vi "rmad event to file.vi"(0 "Skredhendelser":T2(array[cluster]) {"Intensitet terskel 1" format="%.1f"; "Intensitet terskel 2" format="%.1f"; "Intensitet terskel 3" format="%.1f"; "Intensitet terskel 4" format="%.1f"; "Intensitet terskel 5" format="%.1f"}, 1 "vdv_datadir":string, 3 "event_datadir":string, 7 "Recent events 2":T1(array[cluster]) {"SPS" format="%.1f"}, 9 "last packet type":u8[](array[numeric]), 11 "error in":errorcluster, 12 "event to file?":bool[](array[boolean]), 13 "mac adresses":T3) -> (15 "error out":errorcluster)   [LabVIEW 2017]
panel:
  out "previous line in dat file":string
  out "last vdv record number":i32
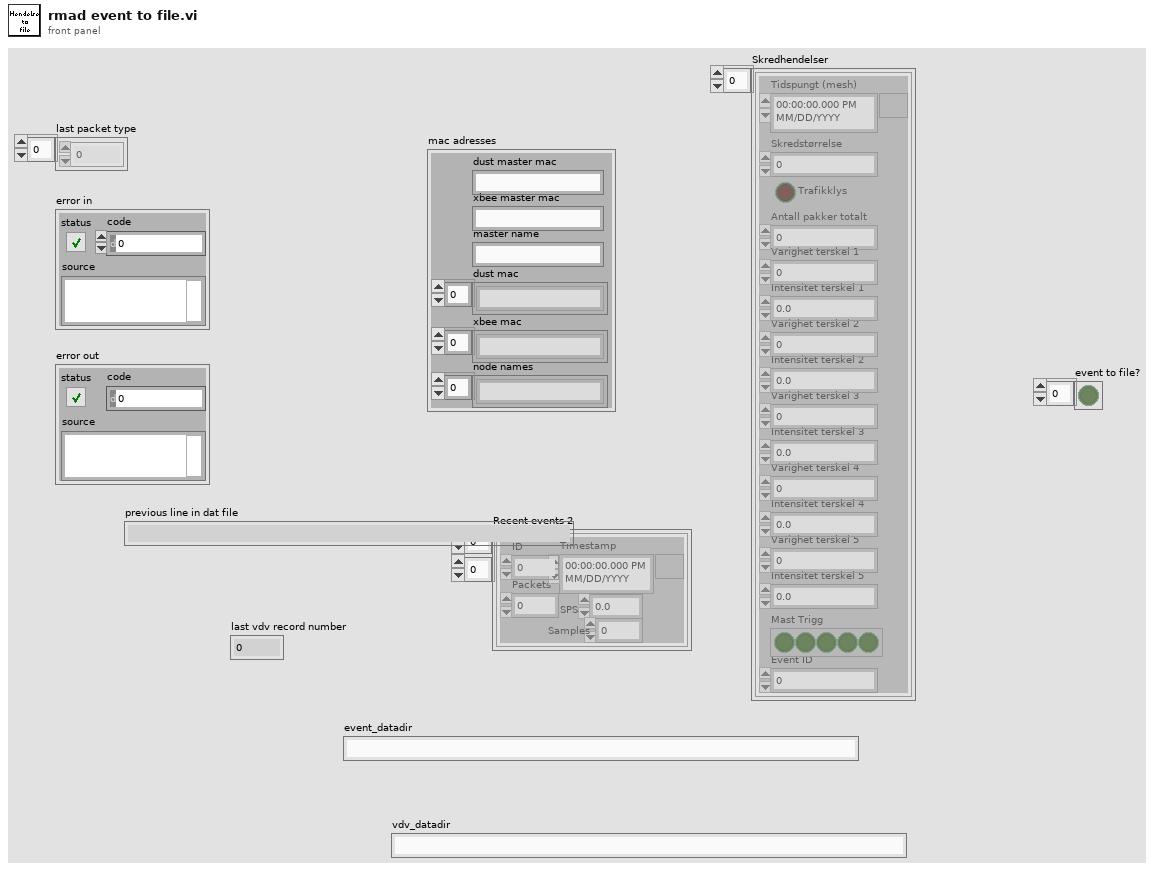
[diagram p1: front panel]
types:
  T1 = cluster{"ID":u16, "Timestamp":timestamp, "Packets":u16, "SPS":dbl, "Samples":u16}[][]
  T2 = cluster{"Tidspungt (mesh)":timestamp, "Skredstørrelse":u16, "Trafikklys":bool, "Antall pakker totalt":u16, "Varighet terskel 1":u16, "Intensitet terskel 1":dbl, "Varighet terskel 2":u16, "Intensitet terskel 2":dbl, "Varighet terskel 3":u16, "Intensitet terskel 3":dbl, "Varighet terskel 4":u16, "Intensitet terskel 4":dbl, "Varighet terskel 5":u16, "Intensitet terskel 5":dbl, "Mast Trigg":bool[], "Event ID":i32}[]
  T3 = cluster{"dust master mac":string, "xbee master mac":string, "master name":string, "dust mac":string[], "xbee mac":string[], "node names":string[]}
  T4 = enum16{"open", "replace", "create", "open or create", "replace or create", "replace or create with confirmation"}
  T5 = cluster{"ID":u16, "Timestamp":timestamp, "Packets":u16, "SPS":dbl, "Samples":u16}
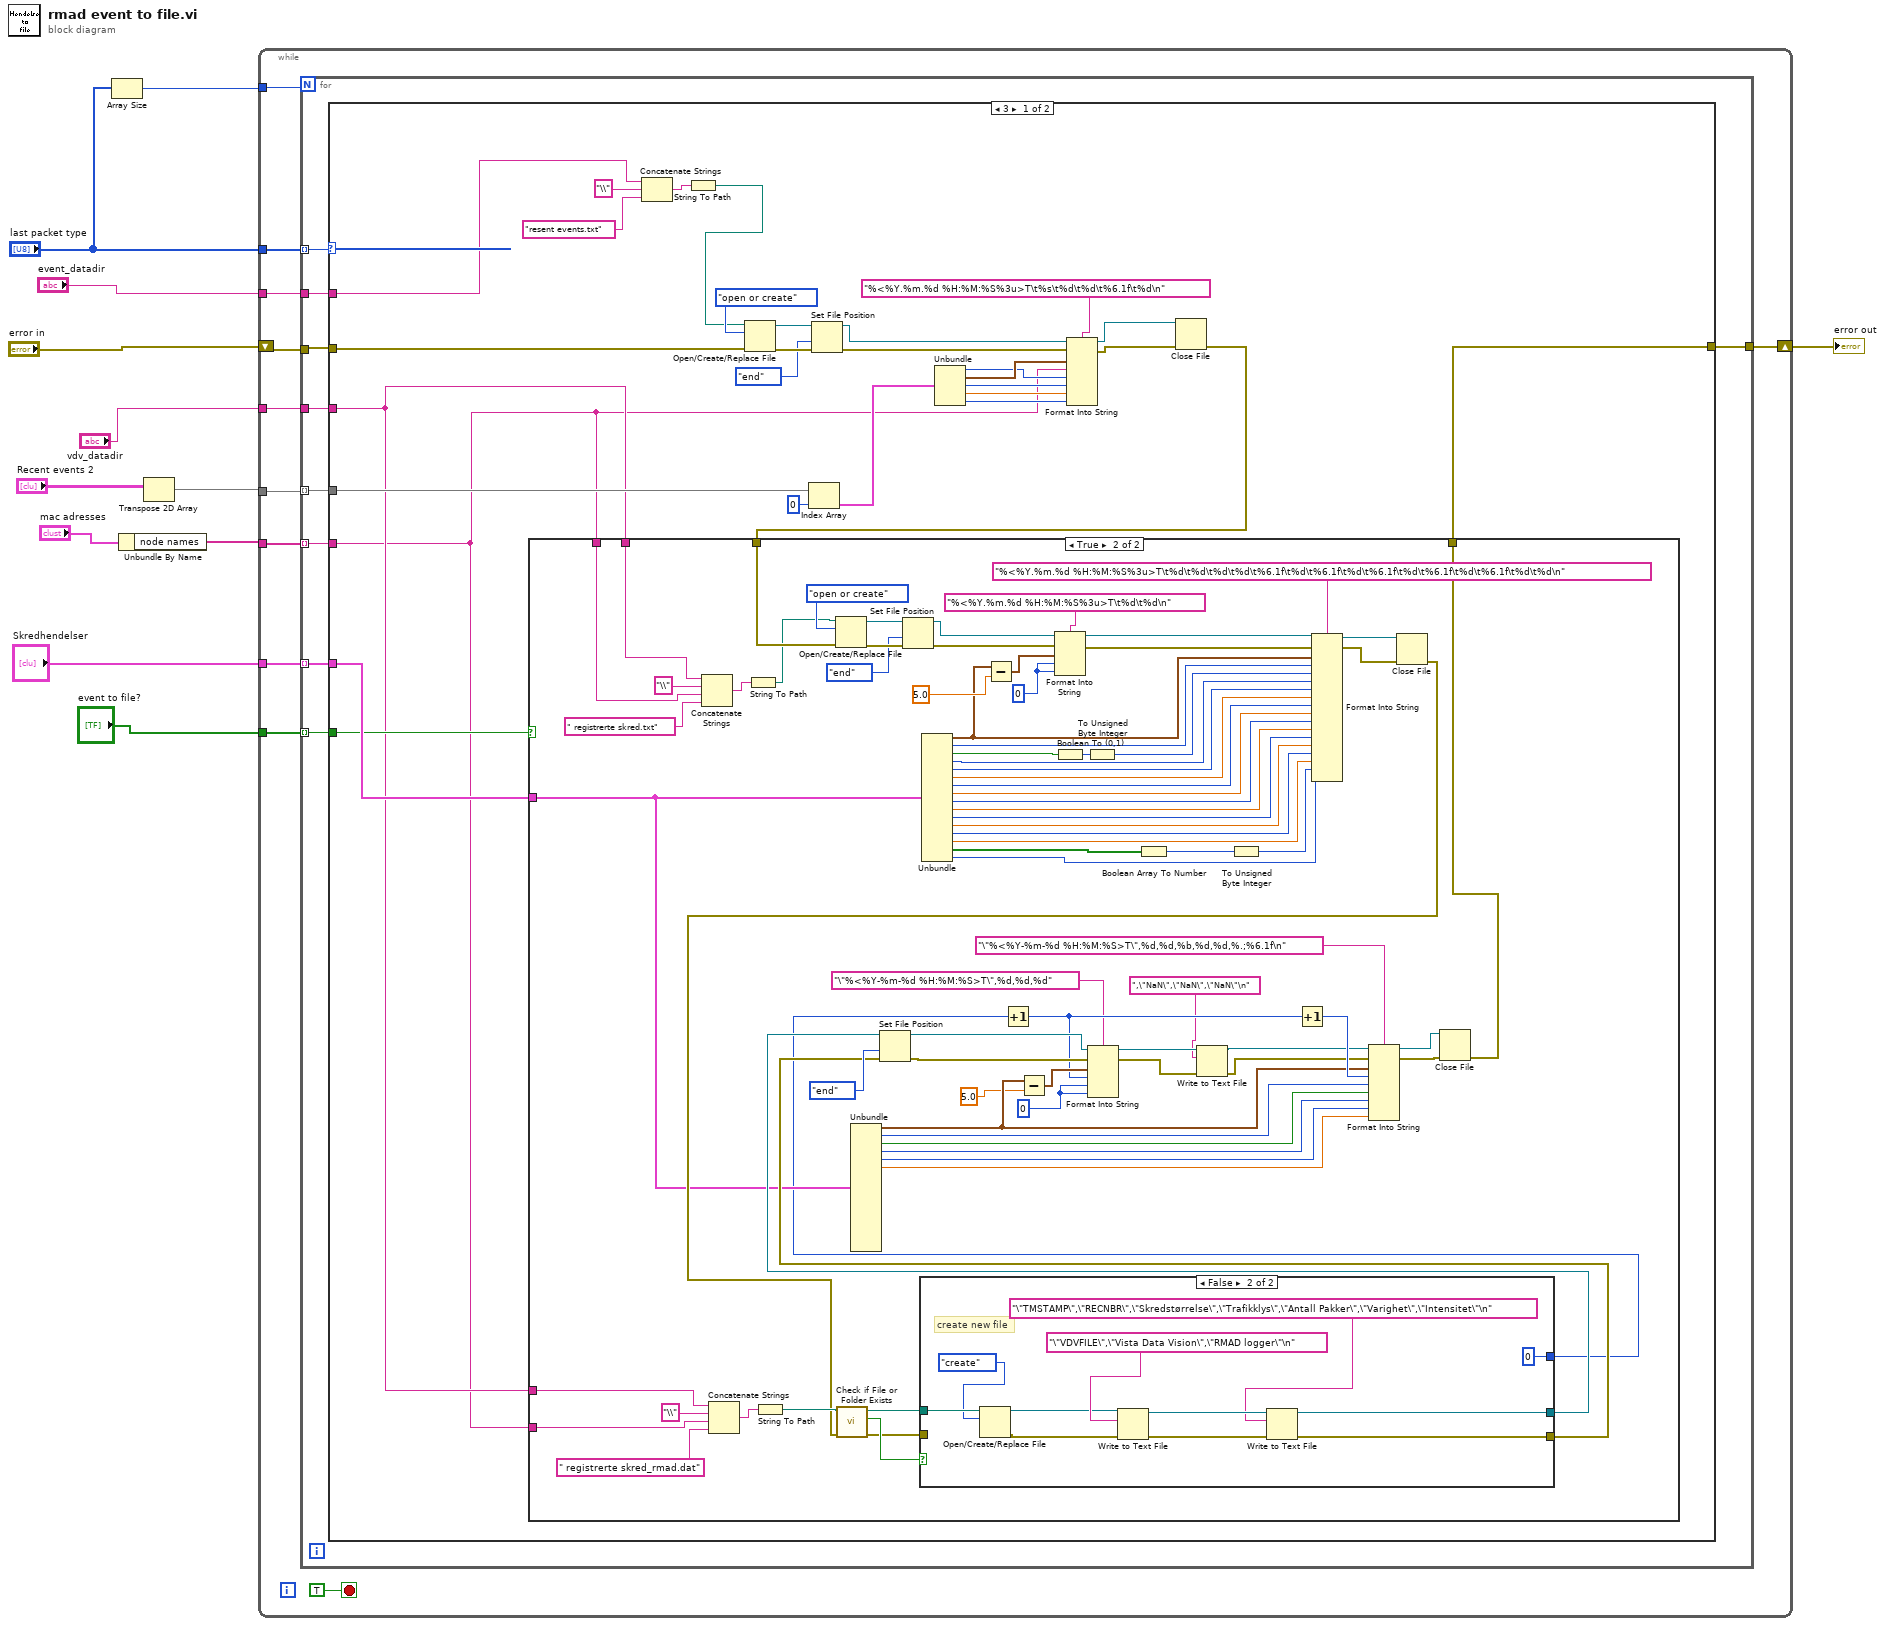
[diagram p0: block diagram]
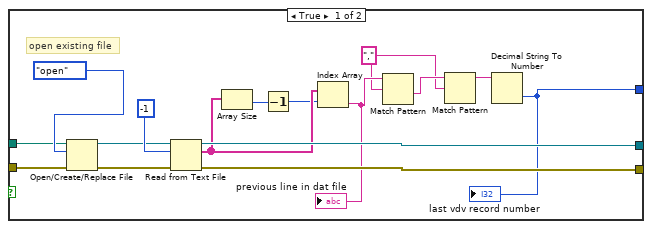
[diagram p3: hidden frame]
diagram:
  n1 = Array Size(array="last packet type") -> (size(s)=w9:i32)
  n2 = Unbundle By Name("mac adresses") -> ("node names"=w6:string[])
  n3 = Transpose 2D Array(2D array="Recent events 2") -> (transposed array=w5:T1)
  n4 = while {
    tunnel: "event_datadir" -> [w21]
    tunnel: w9 -> [w16]
    tunnel: "last packet type" -> [w20]
    tunnel: w6 -> [w19]
    tunnel: w5 -> [w18]
    shift-right: [w22] -> w11
    shift-left: "error in" -> [w23]
    tunnel: "Skredhendelser" -> [w15]
    tunnel: "vdv_datadir" -> [w14]
    tunnel: "event to file?" -> [w13]
    stop <- TRUE stop-if-true
    n5 = for {
      N: w16 -> [_]
      tunnel: w20 -> [w32] mode=indexing
      tunnel: w23 -> [w31]
      tunnel: [w26] -> w22
      tunnel: w21 -> [w30]
      tunnel: w19 -> [w28] mode=indexing
      tunnel: w18 -> [w29] mode=indexing
      tunnel: w15 -> [w27] mode=indexing
      tunnel: w14 -> [w25]
      tunnel: w13 -> [w24] mode=indexing
      n6 = case shown="3" w32 {
        tunnel: w31 -> [w61 w170]
        tunnel: [w39 w170] -> w26
        tunnel: w30 -> [w38 _]
        tunnel: w28 -> [w33 _]
        tunnel: w29 -> [w52 _]
        tunnel: w27 -> [w37 _]
        tunnel: w25 -> [w34 _]
        tunnel: w24 -> [w35 _]
        frame 3 {
          n7 = Concatenate Strings(w38, "\\" ("string"), "resent events.txt" ("string")) -> (w55:string)
          n8 = String To Path(string=w55) -> (path=w54:path)
          n9 = Open/Create/Replace File(file path (use dialog)=w54, error in=w61, operation (0:open)=T4."open or create") -> (refnum out=w58:refnum<file>, error out=w59:errorcluster)  [unwired: 3 in, 1 out]
          n10 = Index Array(array=w52, index=0) -> (element=w50:T5)
          n11 = Set File Position(refnum=w58, from (0:start)=enum16{"start", "end", "current"}."end", error in=w59) -> (refnum out=w43:refnum<file>, error out=w45:errorcluster)  [unwired: 1 in]
          n12 = Unbundle(w50) -> ("ID"=w40:u16, "Timestamp"=w49:timestamp, "Packets"=w48:u16, "SPS"=w36:dbl, "Samples"=w47:u16)
          n13 = Format Into String(format string="%<%Y.%m.%d %H:%M:%S%3u>T\t%s\t%d\t%d\t%6.1f\t%d\n", initial string=w43, error in=w45, w49, w33, w40, w48, w36, w47) -> (resulting string=w42:refnum<file>, error out=w44:errorcluster)
          n14 = Close File(refnum=w42, error in=w44) -> (error out=w41:errorcluster)  [unwired: 1 out]
          n15 = case shown="True" w35 {
            tunnel: w41 -> [w62 w138]
            tunnel: [w62 w83] -> w39
            tunnel: w34 -> [_ w134]
            tunnel: w33 -> [_ w133]
            tunnel: w37 -> [_ w82]
            tunnel: w34 -> [_ w86]
            tunnel: w33 -> [_ w85]
            frame False {
            }
            frame True {
              w71 = u8 0 ("input 2")
              w105 = u8 0 ("input 2")
              n16 = Concatenate Strings(w134, "\\" ("string"), w133, " registrerte skred.txt" ("string")) -> (w136:string)
              n17 = Concatenate Strings(w86, "\\" ("string"), w85, " registrerte skred_rmad.dat" ("string")) -> (w97:string)
              n18 = String To Path(string=w136) -> (path=w132:path)
              n19 = String To Path(string=w97) -> (path=w91:path)
              n20 = Open/Create/Replace File(file path (use dialog)=w132, error in=w138, operation (0:open)=T4."open or create") -> (refnum out=w140:refnum<file>, error out=w141:errorcluster)  [unwired: 3 in, 1 out]
              n21 = Unbundle(w82) -> ("Tidspungt (mesh)"=w73:timestamp, "Skredstørrelse"=w81:u16, "Trafikklys"=w88:bool, "Antall pakker totalt"=w89:u16, "Varighet terskel 1"=w80:u16, "Intensitet terskel 1"=w79:dbl)  [unwired: 10 out]
              n22 = Set File Position(refnum=w140, from (0:start)=enum16{"start", "end", "current"}."end", error in=w141) -> (refnum out=w126:refnum<file>, error out=w128:errorcluster)  [unwired: 1 in]
              n23 = Unbundle(w82) -> ("Tidspungt (mesh)"=w120:timestamp, "Skredstørrelse"=w121:u16, "Trafikklys"=w103:bool, "Antall pakker totalt"=w117:u16, "Varighet terskel 1"=w116:u16, "Intensitet terskel 1"=w115:dbl, "Varighet terskel 2"=w114:u16, "Intensitet terskel 2"=w113:dbl, "Varighet terskel 3"=w112:u16, "Intensitet terskel 3"=w111:dbl, "Varighet terskel 4"=w110:u16, "Intensitet terskel 4"=w109:dbl, "Varighet terskel 5"=w108:u16, "Intensitet terskel 5"=w107:dbl, "Mast Trigg"=w102:bool[], "Event ID"=w104:i32)
              n24 = Subtract(x=w120, y=5.0) -> (x-y=w123:timestamp)
              n25 = Subtract(x=w73, y=5.0) -> (x-y=w76:timestamp)
              n26 = Format Into String(format string="%<%Y.%m.%d %H:%M:%S%3u>T\t%d\t%d\n", initial string=w126, error in=w128, w123, w105, w105) -> (resulting string=w125:refnum<file>, error out=w127:errorcluster)
              n27 = Boolean To (0,1)(Boolean=w103) -> (0, 1=w118:i16)
              n28 = To Unsigned Byte Integer(number=w118) -> (unsigned 8bit integer=w119:u8)
              n29 = Boolean Array To Number(Boolean array=w102) -> (number=w101:u32)
              n30 = To Unsigned Byte Integer(number=w101) -> (unsigned 8bit integer=w106:u8)
              n31 = Format Into String(format string="%<%Y.%m.%d %H:%M:%S%3u>T\t%d\t%d\t%d\t%d\t%6.1f\t%d\t%6.1f\t%d\t%6.1f\t%d\t%6.1f\t%d\t%6.1f\t%d\t%d\n", initial string=w125, error in=w127, w120, w121, w119, w117, w116, w115, w114, w113, w112, w111, w110, w109, w108, w107, w106, w104) -> (resulting string=w129:refnum<file>, error out=w130:errorcluster)
              n32 = Close File(refnum=w129, error in=w130) -> (error out=w84:errorcluster)  [unwired: 1 out]
              n33 = call <vilib>:"Check if File or Folder Exists.vi"("error in (no error)"=w84, "path"=w91) -> ("error out"=w94:errorcluster, "file or folder exists?"=w95:bool, "dup path"=w90:path)  [unwired: 7 in]
              n34 = case shown="False" w95 {
                tunnel: w90 -> [w156 w169]
                tunnel: [w155 w161] -> w93
                tunnel: [w154 w160] -> w92
                tunnel: w94 -> [w158 _]
                tunnel: [w143 0] -> w70
                frame True {
                  w145 = "," ("regular expression")
                  # "open existing file"
                  n35 = Open/Create/Replace File(file path (use dialog)=w156, error in=w158, operation (0:open)=T4."open") -> (refnum out=w151:refnum<file>, error out=w152:errorcluster)  [unwired: 3 in, 1 out]
                  n36 = Read from Text File(file (use dialog)=w151, count=-1, error in=w152) -> (refnum out=w154:refnum<file>, text=w150:string[], error out=w155:errorcluster)  [unwired: 1 in, 1 out]
                  n37 = Array Size(array=w150) -> (size(s)=w149:i32)
                  n38 = Decrement(x=w149) -> (x-1=w148:i32)
                  n39 = Index Array(array=w150, index=w148) -> (element=w147:string)
                  "previous line in dat file" <- w147
                  n40 = Match Pattern(string=w147, regular expression=w145) -> (after substring=w146:string)  [unwired: 1 in, 3 out]
                  n41 = Match Pattern(string=w146, regular expression=w145) -> (before substring=w144:string)  [unwired: 1 in, 3 out]
                  n42 = Decimal String To Number(string=w144) -> (number=w143:i32)  [unwired: 2 in, 1 out]
                  "last vdv record number" <- w143
                }
                frame False {
                  # "create new file"
                  n43 = Open/Create/Replace File(file path (use dialog)=w169, operation (0:open)=T4."create") -> (refnum out=w165:refnum<file>, error out=w166:errorcluster)  [unwired: 4 in, 1 out]
                  n44 = Write to Text File(file (use dialog)=w165, text="\"VDVFILE\",\"Vista Data Vision\",\"RMAD logger\"\n" ("format string"), error in=w166) -> (refnum out=w163:refnum<file>, error out=w164:errorcluster)  [unwired: 1 in, 1 out]
                  n45 = Write to Text File(file (use dialog)=w163, text="\"TMSTAMP\",\"RECNBR\",\"Skredstørrelse\",\"Trafikklys\",\"Antall Pakker\",\"Varighet\",\"Intensitet\"\n" ("format string"), error in=w164) -> (refnum out=w160:refnum<file>, error out=w161:errorcluster)  [unwired: 1 in, 1 out]
                }
              }
              n46 = Set File Position(refnum=w92, from (0:start)=enum16{"start", "end", "current"}."end", error in=w93) -> (refnum out=w74:refnum<file>, error out=w75:errorcluster)  [unwired: 1 in]
              n47 = Increment(x=w70) -> (x+1=w69:i32)
              n48 = Format Into String(format string="\"%<%Y-%m-%d %H:%M:%S>T\",%d,%d,%d", initial string=w74, error in=w75, w76, w69, w71, w71) -> (resulting string=w67:refnum<file>, error out=w65:errorcluster)
              n49 = Write to Text File(file (use dialog)=w67, text=",\"NaN\",\"NaN\",\"NaN\"\n", error in=w65) -> (refnum out=w66:refnum<file>, error out=w64:errorcluster)  [unwired: 1 in, 1 out]
              n50 = Increment(x=w69) -> (x+1=w87:i32)
              n51 = Format Into String(format string="\"%<%Y-%m-%d %H:%M:%S>T\",%d,%d,%b,%d,%d,%.;%6.1f\n", initial string=w66, error in=w64, w73, w87, w81, w88, w89, w80, w79) -> (resulting string=w77:refnum<file>, error out=w78:errorcluster)
              n52 = Close File(refnum=w77, error in=w78) -> (error out=w83:errorcluster)  [unwired: 1 out]
            }
          }
        }
        frame 100, Default {
        }
      }
    }
  }
  "error out" <- w11
